vi "Send Set Delay.vi"(7 "Message Priority (Normal)":T1=enum."Normal", 8 "error in (no error)":errorcluster, 9 "Line":i32, 10 "PWM Delay":dbl format="%.3g", 11 "Message Enqueuer":refnum<class "Message Enqueuer.lvclass">) -> (0 "error out":errorcluster, 3 "Message Enqueuer out":refnum<class "Message Enqueuer.lvclass">)   [LabVIEW 2020, in "BNT_ULx.lvlib" / "Set Delay Msg.lvclass"]
doc: "Sends the <B>BNT_ULx.lvlib:Set Delay Msg.lvclass</B> message.\n\n<B>BNT_DAQmx.lvlib:BNT_DAQmx-MCSV-DOPWM.lvclass:Set Delay.vi</B> Description:\n\nSet pulse delay at index."
uses:
  Set Delay Msg.lvclass
  <vilib>/ActorFramework/Message Enqueuer/Message Enqueuer.lvclass
  <vilib>/ActorFramework/Message Enqueuer/Message Priority.ctl
  C:/Program Files (x86)/National Instruments/LabVIEW 2020/vi.lib/ActorFramework/Message/Message.lvclass
  Set Delay Msg.lvclass/Set Delay Msg.ctl
  <vilib>/ActorFramework/Message Enqueuer/Message Enqueuer.lvclass/Message Enqueuer.ctl
  <vilib>/ActorFramework/Message Priority Queue/Priority Enqueue.vi
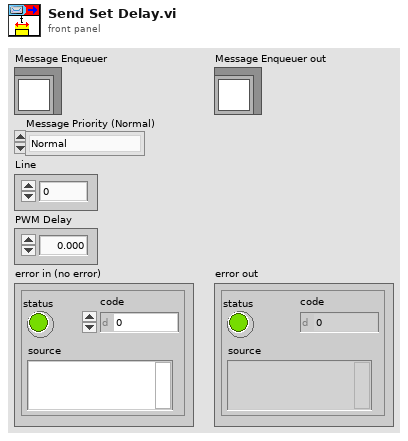
[diagram p1: front panel]
types:
  T1 = typedef "Actor Framework.lvlib/Message Enqueuer.lvclass/Message Priority.ctl" = enum16{"Low", "Normal", "High"}
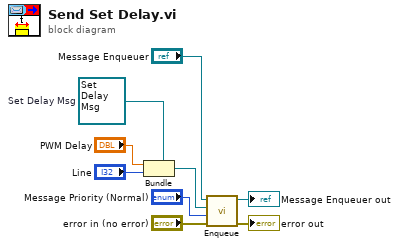
[diagram p0: block diagram]
diagram:
  w3 = refnum<class "Set Delay Msg.lvclass"> refnum  # Set Delay Msg
  n1 = Bundle(cluster=w3, "PWM Delay", "Line") -> (w6:refnum<class "Set Delay Msg.lvclass">)
  n2 = call <vilib>:"Enqueue.vi"("error in (no error)"="error in (no error)", "Message Priority (Normal)"="Message Priority (Normal)", "Message"=w6, "Message Enqueuer in"="Message Enqueuer") -> ("error out"=→"error out":errorcluster, "Message Enqueuer out"=→"Message Enqueuer out":refnum<class "Message Enqueuer.lvclass">)  [unwired: 6 in]
